vi "Capture Video From Camera.vi"() -> ()   [LabVIEW 2018]
doc: "Capture Video From Camera: This example is an example of Capture Video From Camera, which can capture video streams through a camera and display them on the front panel."
uses:
  vi.lib/VIRobotics/opencv_yiku/ctls/ColorConversionCodes.ctl
  vi.lib/VIRobotics/opencv_yiku/Mat/Create_Mat_8U.vi
  vi.lib/VIRobotics/opencv_yiku/Cap/Cap.lvclass
  vi.lib/VIRobotics/opencv_yiku/Mat/Mat_8U/Mat_8U.lvclass
  vi.lib/VIRobotics/opencv_yiku/opencv_yiku.lvlib
panel:
  in  "URL":string="http://192.168.1.42:8000/video"
  in  "Source":enum16{"cameraID", "URL"}(ring)
  in  "cameraID":i32
  out "picture":picture
  in  "stop":bool
  # "Overview: Demonstrates how to capture a video from the camera(USB camera or Webcam) and display it.\nRequirements: Windows.\nInstructions: \n1. Select the Source to use ;\n2. If you select camera,run the VI and you can capture a video from the camera and display it\n3. If you select URL, please fill in the URL with the network camera address.Run the VI and you can capture a video from the camera and display it"
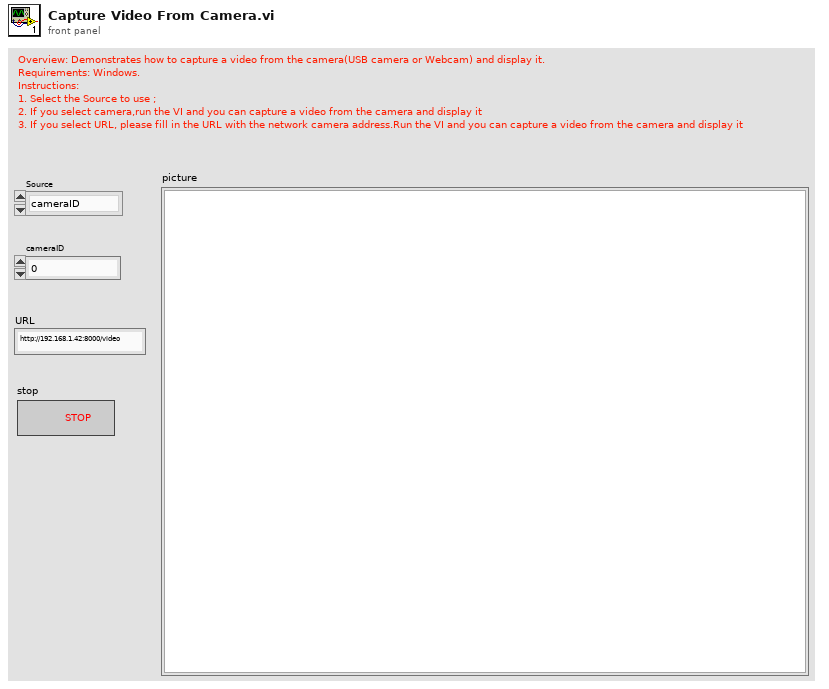
[diagram p1: front panel]
types:
  T1 = typedef "opencv_yiku.lvlib/ColorConversionCodes.ctl" = enum32{"COLOR_BGR2BGRA", "COLOR_BGRA2BGR", "COLOR_BGR2RGBA", "COLOR_RGBA2BGR", "COLOR_BGR2RGB", "COLOR_BGRA2RGBA", "COLOR_BGR2GRAY", "COLOR_RGB2GRAY", "COLOR_GRAY2BGR", "COLOR_GRAY2BGRA", "COLOR_BGRA2GRAY", "COLOR_RGBA2GRAY", "COLOR_BGR2BGR565", "COLOR_RGB2BGR565", "COLOR_BGR5652BGR", "COLOR_BGR5652RGB", "COLOR_BGRA2BGR565", "COLOR_RGBA2BGR565", "COLOR_BGR5652BGRA", "COLOR_BGR5652RGBA", "COLOR_GRAY2BGR565", "COLOR_BGR5652GRAY", "COLOR_BGR2BGR555", "COLOR_RGB2BGR555", "COLOR_BGR5552BGR", "COLOR_BGR5552RGB", "COLOR_BGRA2BGR555", "COLOR_RGBA2BGR555", "COLOR_BGR5552BGRA", "COLOR_BGR5552RGBA", "COLOR_GRAY2BGR555", "COLOR_BGR5552GRAY", "COLOR_BGR2XYZ", "COLOR_RGB2XYZ", "COLOR_XYZ2BGR", "COLOR_XYZ2RGB", "COLOR_BGR2YCrCb", "COLOR_RGB2YCrCb", "COLOR_YCrCb2BGR", "COLOR_YCrCb2RGB", "COLOR_BGR2HSV", "COLOR_RGB2HSV", "42", "43", "COLOR_BGR2Lab", "COLOR_RGB2Lab"}
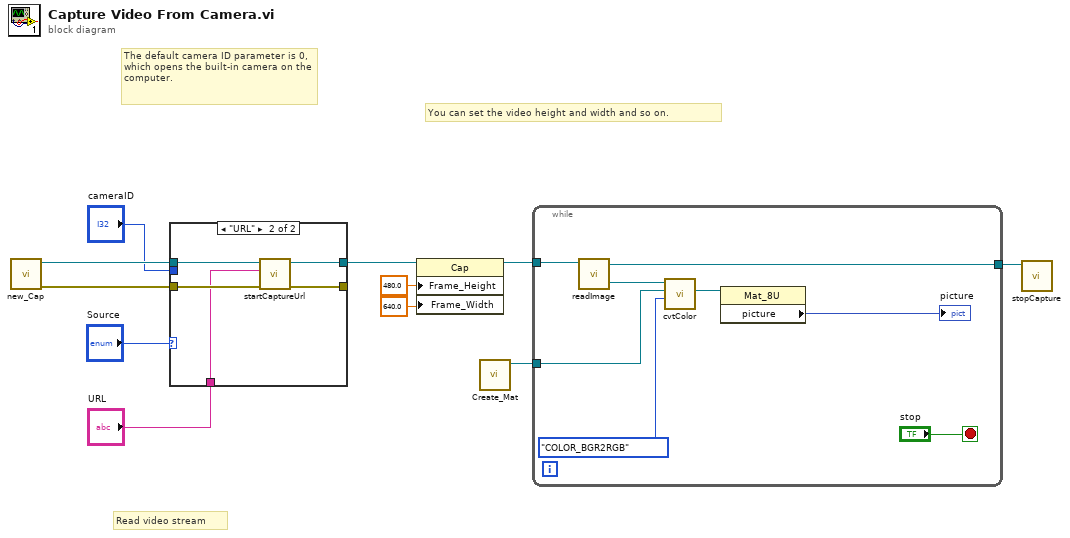
[diagram p0: block diagram]
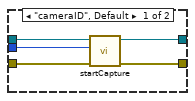
[diagram p2: hidden frame]
diagram:
  # "The default camera ID parameter is 0, which opens the built-in camera on the computer."
  # "Read video stream"
  # "You can set the video height and width and so on."
  n1 = call "new_Cap.vi"() -> ("error out"=w5:errorcluster, "Cap out"=w6:refnum<class "Cap.lvclass">)  [unwired: 10 in]
  n2 = case shown="\"URL\"" "Source" {
    tunnel: w6 -> [w16 w21]
    tunnel: w5 -> [w15 w19]
    tunnel: "cameraID" -> [w14 _]
    tunnel: [w13 w20] -> w1
    tunnel: [w12 w18] -> _
    tunnel: "URL" -> [_ w17]
    frame "cameraID", Default {
      n3 = call "startCapture.vi"("error in (no error)"=w15, "cameraID"=w14, "Cap in"=w16) -> ("error out"=w12:errorcluster, "Cap out"=w13:refnum<class "Cap.lvclass">)  [unwired: 7 in]
    }
    frame "URL" {
      n4 = call-dynamic "startCaptureUrl.vi"("error in (no error)"=w19, "url"=w17, "Cap in"=w21) -> ("error out"=w18:errorcluster, "Cap out"=w20:refnum<class "Cap.lvclass">)  [unwired: 7 in]
    }
  }
  n5 = property class="Cap"(reference=w1, "Frame_Height"=480.0, "Frame_Width"=640.0) -> (reference out=w9:refnum<class "Cap.lvclass">)  [unwired: 1 in, 1 out]
  n6 = call-poly "Create_Mat.vi"() -> ("Mat_8U_out"=w10:refnum<class "Mat_8U.lvclass">)  [unwired: 10 in, 1 out]
  n7 = while {
    tunnel: w9 -> [w29]
    tunnel: [w28] -> w11
    tunnel: w10 -> [w26]
    stop <- "stop" stop-if-true
    n8 = call "readImage.vi"("Cap in"=w29) -> ("Mat out"=w27:refnum<class "Mat_8U.lvclass">, "Cap out"=w28:refnum<class "Cap.lvclass">)  [unwired: 8 in, 1 out]
    n9 = call "cvtColor.vi"("dstCn"=ColorConversionCodes."COLOR_BGR2RGB", "dst"=w26, "src"=w27) -> ("dst out"=w24:refnum<class "Mat_8U.lvclass">)  [unwired: 6 in, 2 out]
    n10 = property class="Mat_8U"(reference=w24) -> ("picture"=→"picture":picture)  [unwired: 1 in, 2 out]
  }
  n11 = call "stopCapture.vi"("Cap in"=w11) -> ()  [unwired: 10 in, 1 out]
